vi "ReadNXTButtonStates.vi"() -> (0 "3 Button Events":enum16{"None", "Pressed", "Released"}[](array[ring]))   [LabVIEW 2012, in "FTC.lvlib" / "Remote Interface.lvlib"]
uses:
  Remote Interface.lvlib
  <vilib>/NXT/Block Support/NXT_ButtonSelector.ctl
panel:
  in  "Oldbuttons":bool[](array[boolean])=[FALSE, FALSE, FALSE]
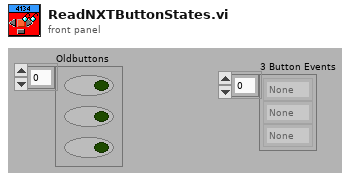
[diagram p1: front panel]
types:
  T1 = typedef "NXT_ButtonSelector.ctl" = u16
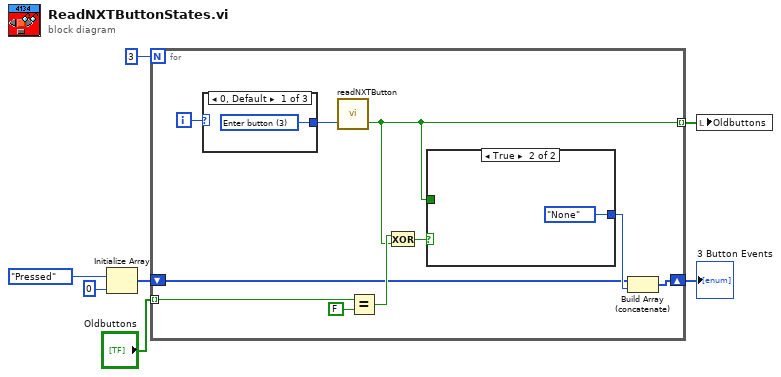
[diagram p0: block diagram]
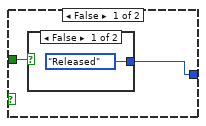
[diagram p2: hidden frame]
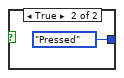
[diagram p3: hidden frame]
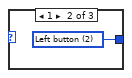
[diagram p4: hidden frame]
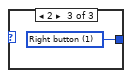
[diagram p5: hidden frame]
diagram:
  n1 = Initialize Array(enum16{"None", "Pressed", "Released"}."Pressed", 0 ("dimension size")) -> (w4:enum16{"None", "Pressed", "Released"}[])
  n2 = for {
    N: 3 -> [_]
    tunnel: "Oldbuttons" -> [w15] mode=indexing
    shift-right: [w9] -> w2
    shift-left: w4 -> [w10]
    tunnel: [w8] -> w1 mode=indexing
    i -> [w17]
    n3 = case shown="0, Default" w17 {
      tunnel: [w23 w24 w25] -> w16
      frame 0, Default {
        w23 = T1 3 items=["Enter button"=3, "Left button"=2, "Right button"=1] ("Button (Enter button)")
      }
      frame 1 {
        w24 = T1 2 items=["Enter button"=3, "Left button"=2, "Right button"=1] ("Button (Enter button)")
      }
      frame 2 {
        w25 = T1 1 items=["Enter button"=3, "Left button"=2, "Right button"=1] ("Button (Enter button)")
      }
    }
    n4 = call <vilib>:"readNXTButton.vi"("Button (Enter button)"=w16) -> ("Yes/No"=w8:bool)  [unwired: 2 in, 1 out]
    n5 = Equal?(x=w15, y=FALSE) -> (x = y?=w12:bool)
    n6 = Exclusive Or(1:w8, 2:w12) -> (0:w13:bool)
    n7 = case shown="True" w13 {
      tunnel: [w18 enum16{"None", "Pressed", "Released"}."None"] -> w11
      tunnel: w8 -> [w19 _]
      frame False {
        n8 = case shown="False" w19 {
          tunnel: [enum16{"None", "Pressed", "Released"}."Released" enum16{"None", "Pressed", "Released"}."Pressed"] -> w18
          frame False {
          }
          frame True {
          }
        }
      }
      frame True {
      }
    }
    n9 = Build Array (concatenate)(w10, w11) -> (w9:enum16{"None", "Pressed", "Released"}[])
  }
  "3 Button Events" <- w2
  n10 = local write "Oldbuttons"(w1) -> ()
